vi "mono-Isconnected.vi"(8 "error in (no error)":errorcluster, 11 "Monochromator":refnum<vi>) -> (0 "error out":errorcluster, 2 "Connected":bool, 3 "Monochromator out":refnum<vi>)   [LabVIEW 2016]
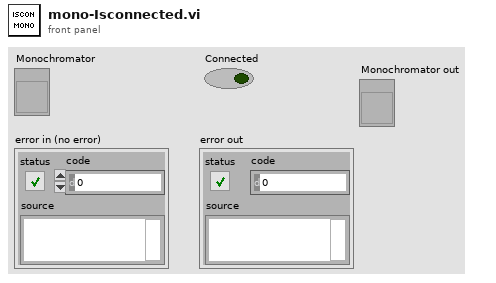
[diagram p1: front panel]
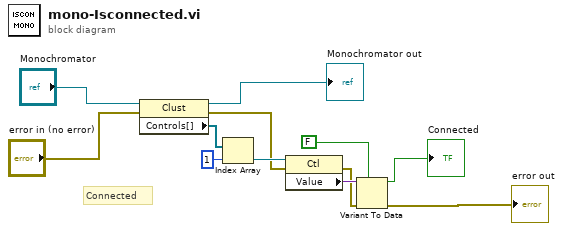
[diagram p0: block diagram]
diagram:
  # "Connected"
  n1 = property class="Clust"(reference="Monochromator", error in="error in (no error)") -> (reference out=→"Monochromator out":refnum<vi>, error out=w5:errorcluster, "Controls[]"=w8:refnum<vi>[])
  n2 = Index Array(array=w8, index=1) -> (element=w6:refnum<vi>)
  n3 = property class="Ctl"(reference=w6, error in=w5) -> (error out=w3:errorcluster, "Value"=w4:variant)  [unwired: 1 out]
  n4 = Variant To Data(error in=w3, type=FALSE, Variant=w4) -> (data=→"Connected":bool, error out=→"error out":errorcluster)
